vi "Create NI 9375.vi"(8 "error in":errorcluster, 11 "channel settings":T1[](array[typedef])) -> (0 "error out":errorcluster, 3 "NI 9375 out":refnum<class "NI 9375.lvclass">)   [LabVIEW 2017, in "Scan Engine Scripting.lvlib" / "NI 9375.lvclass"]
uses:
  NI 9375.lvclass
  Mode Classes/Controls/digital channel settings.ctl
  Mode Classes/Digital Input and Output Mode/Digital Input and Output Mode.lvclass
  C:/dev/niveristand-scan-engine-ethercat-custom-device/Custom Device Source/Scripting/Modules/Mode Classes/Mode/Mode.lvclass
  09133c77-b8c8-4b85-bcb4-a501a172f880.vi
  Scan Engine Scripting.lvlib
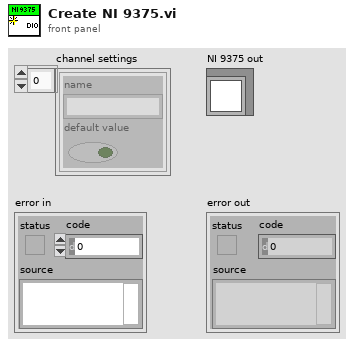
[diagram p1: front panel]
types:
  T1 = typedef "Scan Engine Scripting.lvlib/digital channel settings.ctl" = cluster{"name":string, "default value":bool}
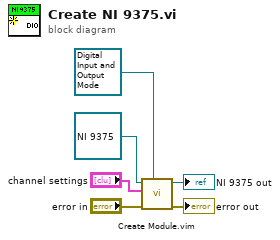
[diagram p0: block diagram]
diagram:
  n1 = call "Create Module.vim"("mode in"=refnum<class "Digital Input and Output Mode.lvclass"> refnum ("Scan Engine Scripting.lvlib:Digital Input and Output Mode.lvclass"), "error in"="error in", "channel settings"="channel settings", "module in"=refnum<class "NI 9375.lvclass"> refnum ("NI 9375 in")) -> ("error out"=→"error out":errorcluster, "module out"=→"NI 9375 out":refnum<class "NI 9375.lvclass">)  [unwired: 6 in]
